vi "Get Todo Bookmarks.vi"(6 "open VI references? (False)":bool, 8 "error in (no error)":errorcluster, 11 "Directory to Search":path) -> (0 "error out":errorcluster, 2 "todo bookmarks":map{path, T1}(c390))   [LabVIEW 2020]
uses:
  <vilib>/Utility/miscctls.llb/LVBookmarkInfoTypeDef.ctl
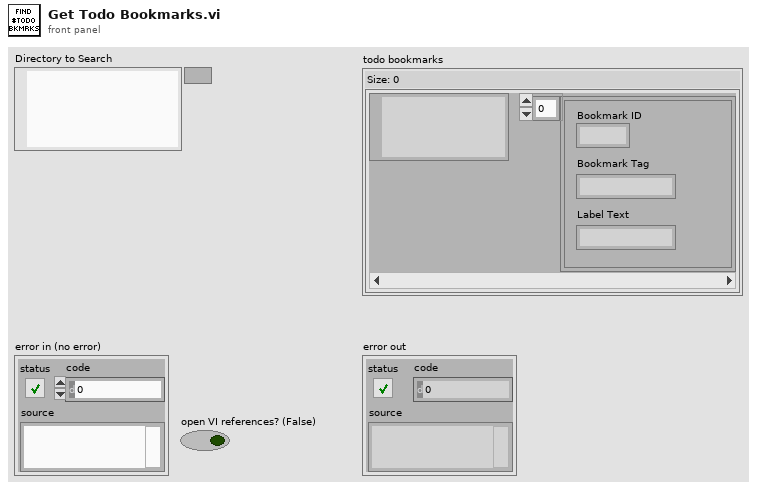
[diagram p1: front panel]
types:
  T1 = typedef "LVBookmarkInfoTypeDef.ctl" = cluster{"Bookmark ID":u32, "Bookmark Tag":string, "Label Text":string}[]
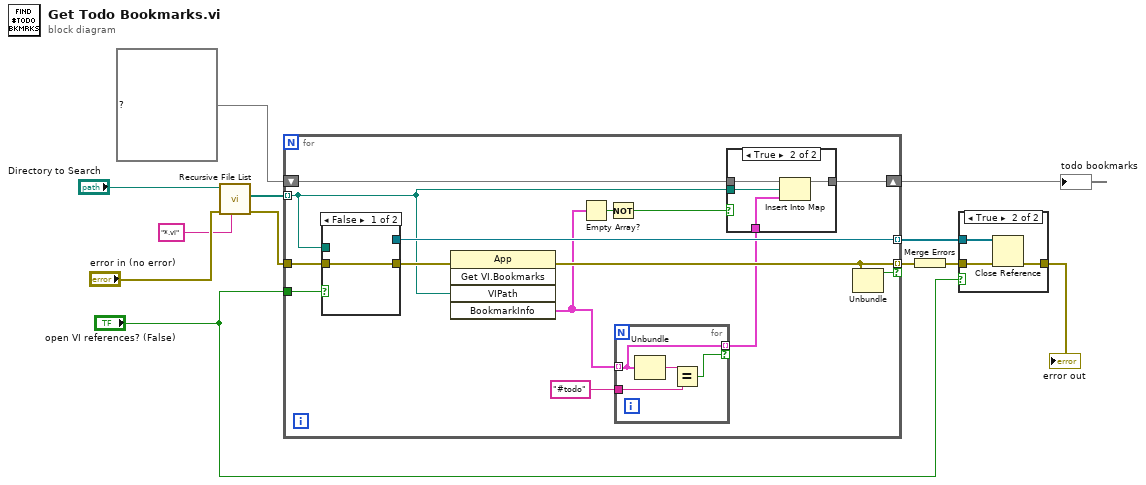
[diagram p0: block diagram]
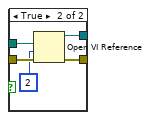
[diagram p3: hidden frame]
diagram:
  n1 = call <vilib>:"Recursive File List.vi"("pattern"="*.vi", "error in (no error)"="error in (no error)", "Folder Path"="Directory to Search") -> ("error out"=w10:errorcluster, "All Files in Dir"=w5:path[])  [unwired: 4 in, 3 out]
  n2 = for {
    tunnel: w5 -> [w22] mode=indexing
    tunnel: [w25] -> w6 mode=indexing
    shift-right: [w23] -> w12
    shift-left: map{path, T1} {} ("empty map") -> [w16]
    tunnel: w10 -> [w24]
    tunnel: [w20] -> w7 mode=indexing if=w19
    tunnel: "open VI references? (False)" -> [w13]
    n3 = case shown="False" w13 {
      tunnel: [w27 w32] -> w26
      tunnel: [_ w31] -> w25
      tunnel: w24 -> [w27 w30]
      tunnel: w22 -> [_ w28]
      frame False {
      }
      frame True {
        n4 = Open VI Reference(vi path=w28, options=2, error in (no error)=w30) -> (vi reference=w31:refnum<vi>, error out=w32:errorcluster)  [unwired: 3 in]
      }
    }
    n5 = invoke class="App" method="Get VI.Bookmarks"(error in=w26, "VIPath"=w22) -> (error out=w20:errorcluster, "BookmarkInfo"=w15:T1)  [unwired: 3 in, 3 out]
    n6 = Empty Array?(array=w15) -> (empty?=w21:bool)
    n7 = Not(x=w21) -> (.not. x?=w18:bool)
    n8 = for {
      tunnel: w15 -> [w34] mode=indexing
      tunnel: "#todo" ("Bookmark Tag") -> [w35]
      tunnel: [w34] -> w14 mode=indexing if=w33
      n9 = Unbundle(w34) -> ("Bookmark Tag"=w36:string)  [unwired: 2 out]
      n10 = Equal?(x=w36, y=w35) -> (x = y?=w33:bool)
    }
    n11 = case shown="True" w18 {
      tunnel: w16 -> [w37 w41]
      tunnel: [w37 w40] -> w23
      tunnel: w22 -> [_ w39]
      tunnel: w14 -> [_ w38]
      frame False {
      }
      frame True {
        n12 = Insert Into Map(map in=w41, key=w39, value=w38) -> (map out=w40:map{path, T1})  [unwired: 2 out]
      }
    }
    n13 = Unbundle(w20) -> ("status"=w19:bool)  [unwired: 2 out]
  }
  "todo bookmarks" <- w12
  n14 = Merge Errors(w7) -> (w9:errorcluster)
  n15 = case shown="True" "open VI references? (False)" {
    tunnel: w9 -> [w42 w45]
    tunnel: [w42 w44] -> w8
    tunnel: w6 -> [_ w43]
    frame False {
    }
    frame True {
      n16 = Close Reference(reference=w43, error in (no error)=w45) -> (error out=w44:errorcluster)
    }
  }
  "error out" <- w8
